vi "(SubVI)Serial_Write.vi"(7 "Echo Request":bool, 8 "error in (no error)":errorcluster caption="에러 입력(에러 없음)", 11 "Data to Write":u8[](array[numeric])) -> (0 "error out":errorcluster caption="에러 출력")   [LabVIEW 2020]
uses:
  Controls/(Ctrl)Serial_FGV Function.ctl
  Variables/(Var)System Variables.vi
panel:
  # "(SubVI)Serial_Write.vi By hspark\n\nDescription : 시리얼 통신 쓰기 VI\n\nInput : \n1. Data to Write : U8 배열의 쓰기할 데이터 입력. Header는 코드에서 생성되므로 Header를 제외한 순수 Data만 입력.\n2. Echo Request : Board로부터 Response가 필요한지 여부. 프로토콜 명시됨.\n\nOutput : \n\nLabVIEW Version : 2020 SP1 이상\n\nNote :\n\nUpdate : 2021.10.06"
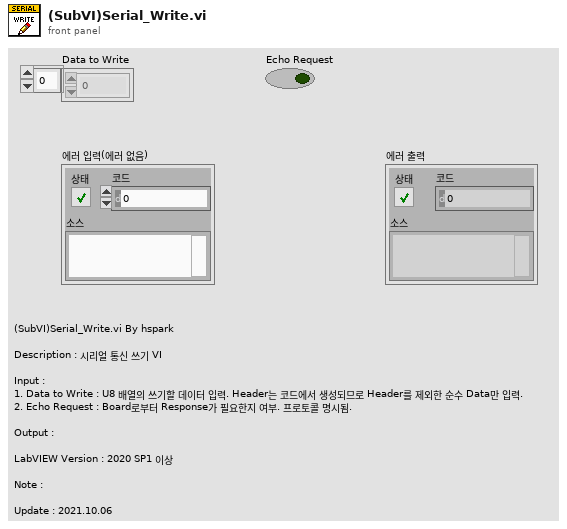
[diagram p1: front panel]
types:
  T1 = typedef "(Ctrl)Serial_FGV Function.ctl" = enum16{"Initialize", "Read", "Read All", "Write", "Flush Buffer", "Get Ref.", "Close"}
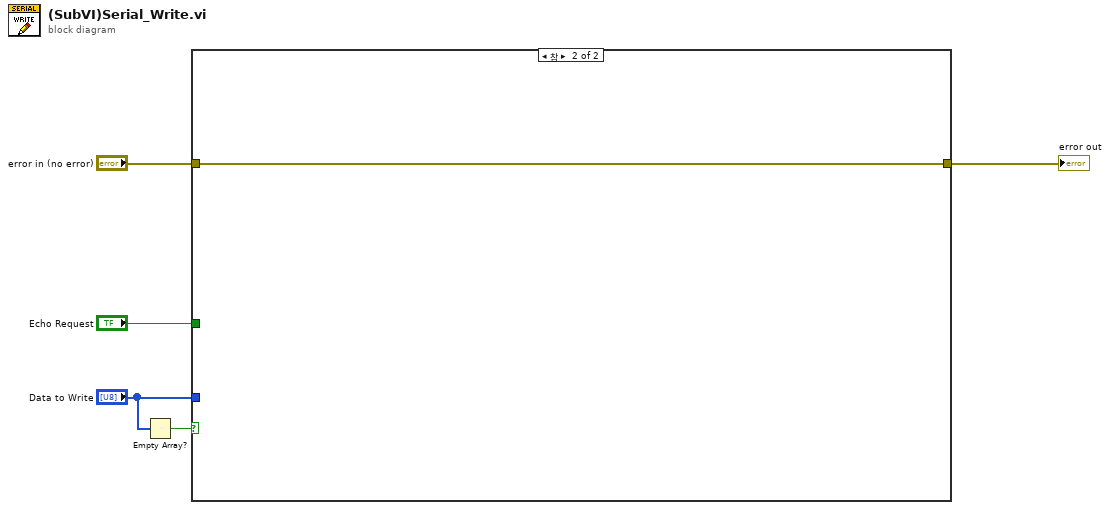
[diagram p0: block diagram]
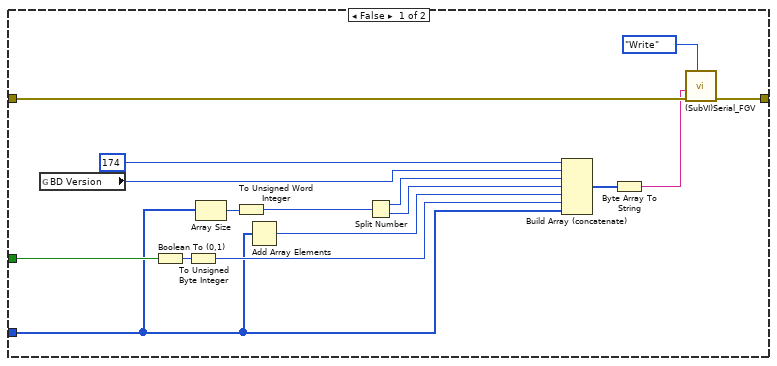
[diagram p2: hidden frame]
diagram:
  n1 = Empty Array?(array="Data to Write") -> (empty?=w1:bool)
  n2 = case shown="참" w1 {
    tunnel: "error in (no error)" -> [w19 w22]
    tunnel: [w18 w22] -> w4
    tunnel: "Echo Request" -> [w10 _]
    tunnel: "Data to Write" -> [w6 _]
    frame False {
      n3 = global read "(Var)System Variables.vi" "BD Version"() -> (w16:u8)
      n4 = Boolean To (0,1)(Boolean=w10) -> (0, 1=w9:i16)
      n5 = To Unsigned Byte Integer(number=w9) -> (unsigned 8bit integer=w21:u8)
      n6 = Array Size(array=w6) -> (size(s)=w15:i32)
      n7 = To Unsigned Word Integer(number=w15) -> (unsigned 16bit integer=w14:u16)
      n8 = Add Array Elements(numeric array=w6) -> (sum=w11:u8)
      n9 = Split Number(x=w14) -> (hi(x)=w13:u8, lo(x)=w12:u8)
      n10 = Build Array (concatenate)(u8 174 ("숫자형"), w16, w13, w12, w11, w21, w6) -> (w8:u8[])
      n11 = Byte Array To String(unsigned byte array=w8) -> (string=w7:string)
      n12 = call "(SubVI)Serial_FGV.vi"("Function"=(Ctrl)Serial_FGV_Function."Write", "error in (no error)"=w19, "Data to Write"=w7) -> ("error out"=w18:errorcluster)  [unwired: 6 in, 2 out]
    }
    frame True {
    }
  }
  "error out" <- w4
